vi "check_timeout.vi"(8 "error in":errorcluster, 11 "Timeout?":bool) -> (0 "error out":errorcluster)   [LabVIEW 2011, in "Fiberscope_library.lvlib"]
uses:
  Fiberscope_library.lvlib
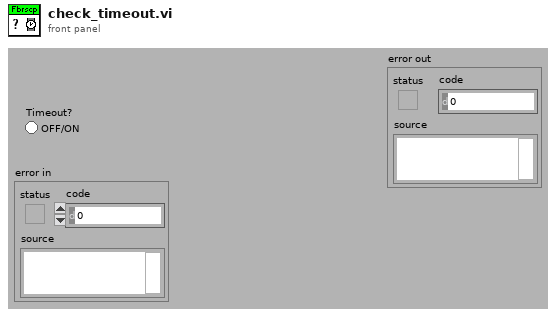
[diagram p1: front panel]
types:
  T1 = cluster{"error in (no error)":errorcluster, string}
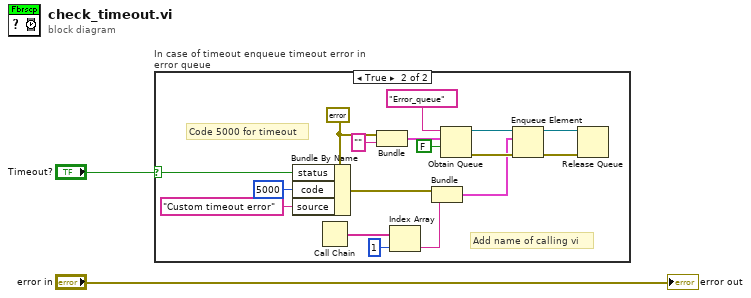
[diagram p0: block diagram]
diagram:
  n1 = case "In case of timeout enqueue timeout error in error queue" shown="True" "Timeout?" {
    selector: "Timeout?" -> [_ w3]
    frame False {
    }
    frame True {
      w4 = errorcluster {"status"=FALSE, "code"=0, "source"=""} ("error in (no error)")
      # "Code 5000 for timeout"
      # "Add name of calling vi"
      n2 = Bundle By Name(cluster=w4, "status"=w3, "code"=5000, "source"="Custom timeout error") -> (w8:errorcluster)
      n3 = Call Chain() -> (call chain=w13:string[])
      n4 = Bundle("error in (no error)"=w4, "") -> (w10:T1)  [unwired: 1 in]
      n5 = Index Array(array=w13, index=1) -> (element=w6:string)
      n6 = Bundle("error in (no error)"=w8, w6) -> (w7:T1)  [unwired: 1 in]
      n7 = Obtain Queue(name (unnamed)="Error_queue", element data type=w10, create if not found? (T)=FALSE) -> (queue out=w18:refnum<queue>, error out=w16:errorcluster)  [unwired: 2 in, 1 out]
      n8 = Enqueue Element(queue=w18, element=w7, error in (no error)=w16) -> (queue out=w17:refnum<queue>, error out=w15:errorcluster)  [unwired: 1 in, 1 out]
      n9 = Release Queue(queue=w17, error in (no error)=w15) -> ()  [unwired: 1 in, 3 out]
    }
  }
  "error out" <- "error in"
